vi "RProp Update.vi"(8 "Teaching Coef In":T1[](array[typedef]), 9 "Previous Gradient In":T1[](array[typedef]), 10 "Current Gradient In":T1[](array[typedef]), 11 "Neural Network In":T2) -> (1 "Teaching Coef Out":T1[](array[typedef]), 2 "Gradient Out":T1[](array[typedef]), 3 "Neural Network Out":T2)   [LabVIEW 2011, in "Super Simple Neural Network.lvlib"]
uses:
  Super Simple Neural Network.lvlib
  Types/2D Array.ctl
  Types/Neural Network.ctl
  Types/Scaling Info.ctl
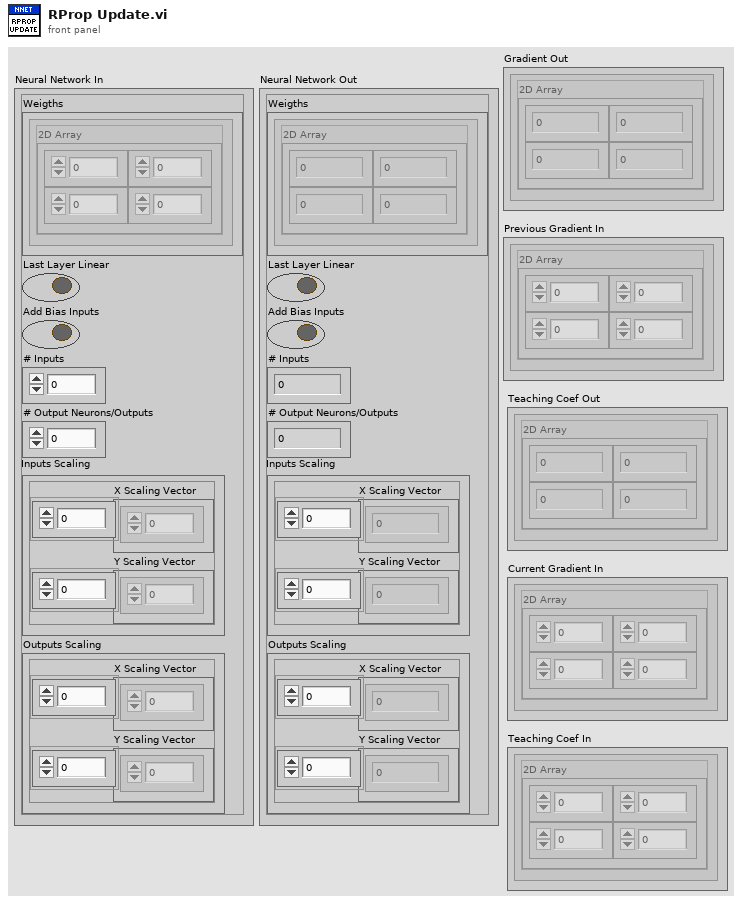
[diagram p1: front panel]
types:
  T1 = typedef "Super Simple Neural Network.lvlib/2D Array.ctl" = cluster{"2D Array":dbl[][]}
  T2 = typedef "Super Simple Neural Network.lvlib/Neural Network.ctl" = cluster{"Weigths":T1[], "Last Layer Linear":bool, "Add Bias Inputs":bool, "# Inputs":u32, "# Output Neurons/Outputs":u32, "Inputs Scaling":T3, "Outputs Scaling":T3}
  T3 = typedef "Super Simple Neural Network.lvlib/Scaling Info.ctl" = cluster{"X Scaling Vector":dbl[], "Y Scaling Vector":dbl[]}
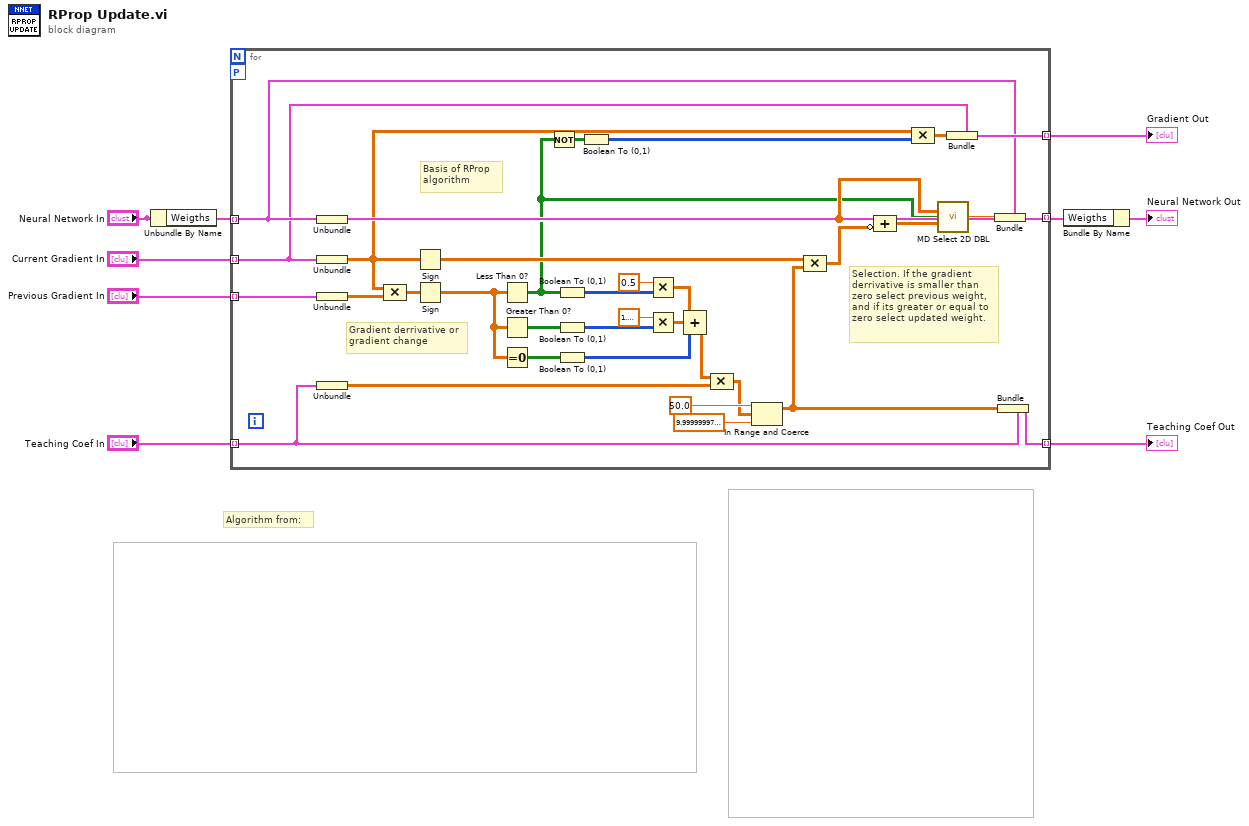
[diagram p0: block diagram]
diagram:
  # "Algorithm from:"
  n1 = Unbundle By Name("Neural Network In") -> ("Weigths"=w1:T1[])
  n2 = for {
    tunnel: w1 -> [w16] mode=indexing
    tunnel: [w44] -> w2 mode=indexing
    tunnel: "Current Gradient In" -> [w17] mode=indexing
    tunnel: "Previous Gradient In" -> [w43] mode=indexing
    tunnel: "Teaching Coef In" -> [w14] mode=indexing
    tunnel: [w42] -> w4 mode=indexing
    tunnel: [w41] -> w5 mode=indexing
    workers-P: _ -> [_]
    # "Selection. If the gradient\nderrivative is smaller than\nzero select previous weight,\nand if its greater or equal to\nzero select updated weight."
    # "Basis of RProp \nalgorithm"
    # "Gradient derrivative or\ngradient change"
    # "Iterate over the layers of the network and update the weigths"
    n3 = Unbundle(w16) -> ("2D Array"=w13:dbl[][])
    n4 = Unbundle(w17) -> ("2D Array"=w23:dbl[][])
    n5 = Unbundle(w43) -> ("2D Array"=w26:dbl[][])
    n6 = Unbundle(w14) -> ("2D Array"=w38:dbl[][])
    n7 = Compound Arithmetic op=MULTIPLY(w23, w26) -> (w33:dbl[][])
    n8 = Sign(1:w23) -> (0:w25:dbl[][])
    n9 = Sign(1:w33) -> (0:w35:dbl[][])
    n10 = Less Than 0?(x=w35) -> (x < 0?=w10:bool[][])
    n11 = Greater Than 0?(x=w35) -> (x > 0?=w40:bool[][])
    n12 = Equal To 0?(x=w35) -> (x = 0?=w29:bool[][])
    n13 = Not(x=w10) -> (.not. x?=w28:bool[][])
    n14 = Boolean To (0,1)(Boolean=w10) -> (0, 1=w15:i16[][])
    n15 = Boolean To (0,1)(Boolean=w40) -> (0, 1=w39:i16[][])
    n16 = Boolean To (0,1)(Boolean=w29) -> (0, 1=w30:i16[][])
    n17 = Boolean To (0,1)(Boolean=w28) -> (0, 1=w21:i16[][])
    n18 = Multiply(x=0.5, y=w15) -> (x*y=w19:dbl[][])
    n19 = Multiply(x=1.2000000476837158, y=w39) -> (x*y=w18:dbl[][])
    n20 = Compound Arithmetic op=ADD(w19, w18, w30) -> (w34:dbl[][])
    n21 = Compound Arithmetic op=MULTIPLY(w34, w38) -> (w24:dbl[][])
    n22 = In Range and Coerce(upper limit=50.0, x=w24, lower limit=9.999999974752427e-07) -> (coerced(x)=w20:dbl[][])  [unwired: 1 out]
    n23 = Compound Arithmetic op=MULTIPLY(w25, w20) -> (w27:dbl[][])
    n24 = Compound Arithmetic op=ADD(w13, invert w27) -> (w12:dbl[][])
    n25 = Compound Arithmetic op=MULTIPLY(w23, w21) -> (w22:dbl[][])
    n26 = call "MD Select 2D DBL.vi"("First Array"=w13, "Condition"=w10, "Second Array"=w12) -> ("Resulting Array"=w11:dbl[][])  [unwired: 12 in]
    n27 = Bundle(cluster=w17, "2D Array"=w22) -> (w41:T1)
    n28 = Bundle(cluster=w16, "2D Array"=w11) -> (w44:T1)
    n29 = Bundle(cluster=w14, "2D Array"=w20) -> (w42:T1)
  }
  "Gradient Out" <- w5
  "Teaching Coef Out" <- w4
  n30 = Bundle By Name(cluster="Neural Network In", "Weigths"=w2) -> (→"Neural Network Out":T2)
